vi "BackupSettings.vi"() -> ()   [LabVIEW 2022 SP3]
panel:
  out "SettingsPath":path
  out "error out":errorcluster
  out "Generated Zip File":path
  out "DataPath":path
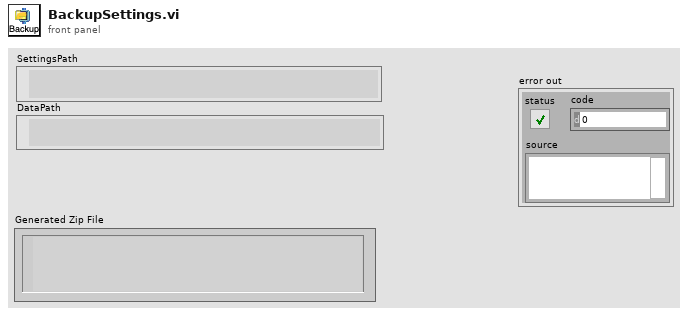
[diagram p1: front panel]
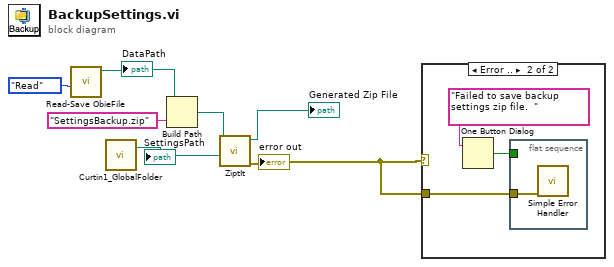
[diagram p0: block diagram]
diagram:
  n1 = call "Read-Save ObieFile.vi"("Task"=enum16{"Save", "Read"}."Read") -> ("DataPath Out"=w5:path)  [unwired: 8 in, 2 out]
  "DataPath" <- w5
  n2 = call "Curtin1_GlobalFolder.vi"() -> ("LabVIEW Data Path"=w2:path)  [unwired: 1 in, 1 out]
  "SettingsPath" <- w2
  n3 = Build Path(base path=w5, name or relative path="SettingsBackup.zip") -> (appended path=w6:path)
  n4 = call "ZiptIt.vi"("Folder to zip"=w2, "Zip file"=w6) -> ("error out"=w1:errorcluster, "Generated Zip File"=→"Generated Zip File":path)  [unwired: 8 in]
  "error out" <- w1
  n5 = case shown="Error .." w1 {
    tunnel: w1 -> [_ w9]
    frame No Error {
    }
    frame Error {
      n6 = One Button Dialog(message="Failed to save backup settings zip file.  ") -> (true=w8:bool)  [unwired: 1 in]
      n7 = flat-sequence {
        tunnel: w9 -> [w11]
        tunnel: w8 -> [_]
        frame #0 {
          n8 = call <vilib>:"Simple Error Handler.vi"("error in (no error)"=w11) -> ()  [unwired: 4 in, 5 out]
        }
      }
    }
  }
